vi "VI前面板截图.vi"(8 "矩形边界":T1 caption="子矩形", 11 "被绘图VI":refnum<vi>) -> (0 "错误输出":errorcluster, 2 "image subset":T2 caption="图像子集", 3 "new picture":picture caption="新图片")   [LabVIEW 2017]
doc: "获取VI截图或部分截图，矩形输入空则为全面版截图。"
uses:
  <vilib>/picture/picture.llb/imagedata.ctl
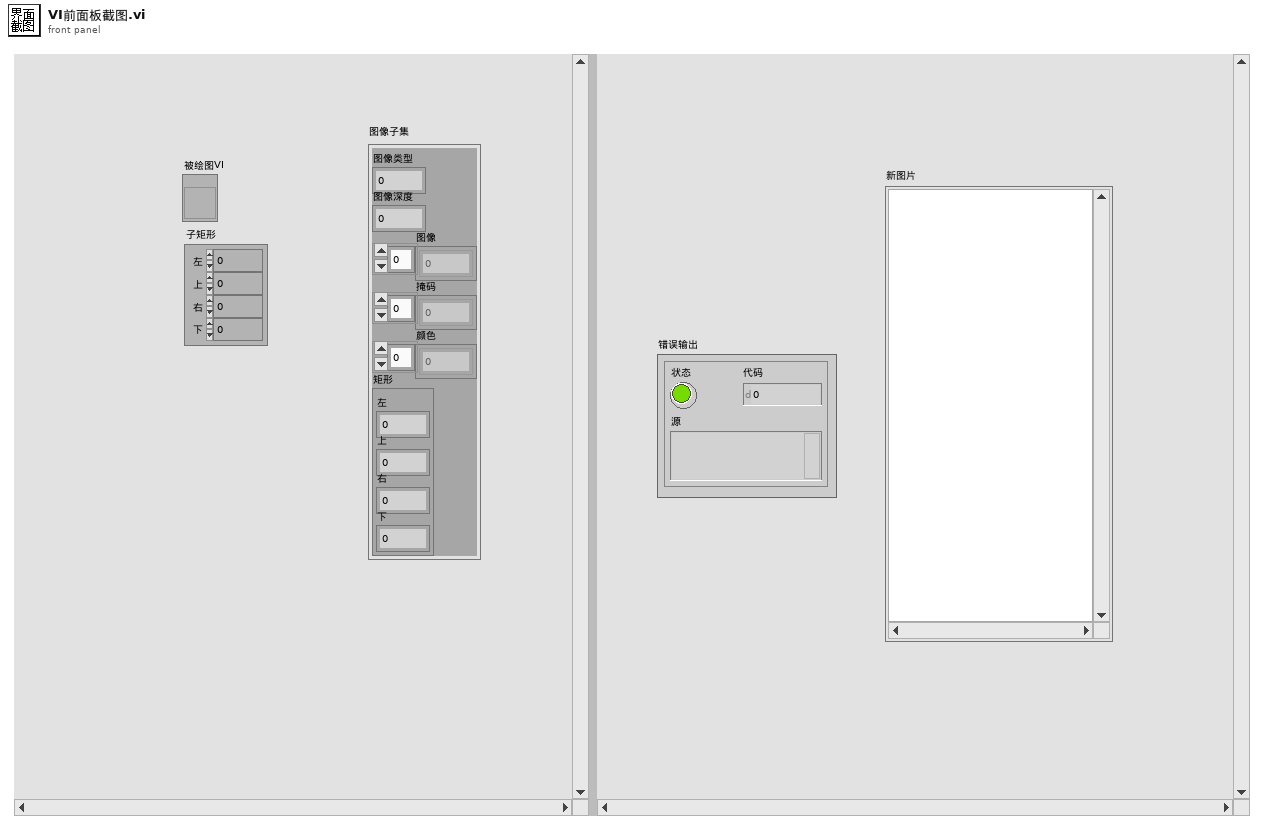
[diagram p1: front panel]
types:
  T1 = cluster{"left":i16, "top":i16, "right":i16, "bottom":i16}
  T2 = typedef "imagedata.ctl" = cluster{"image type":i32, "image depth":i32, "image":u8[], "mask":u8[], "colors":u32[], "Rectangle":cluster{"left":i16, "top":i16, "right":i16, "bottom":i16}}
  T3 = cluster{"left":bool, "top":bool, "right":bool, "bottom":bool}
  T4 = typedef "LVRectTypeDef.ctl" = cluster{"Left":i16, "Top":i16, "Right":i16, "Bottom":i16}
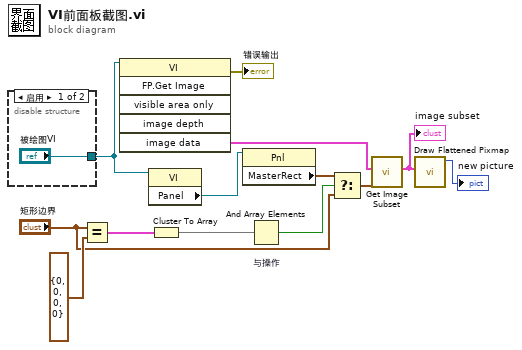
[diagram p0: block diagram]
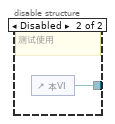
[diagram p2: hidden frame]
diagram:
  n1 = disable-structure shown="启用" {
    disable-tunnel: ["被绘图VI" w15] -> w6
    frame Enabled {
    }
    frame Disabled {
      # "测试使用"
      n2 = control-ref of="本VI"() -> (w15:refnum<vi>)
    }
  }
  n3 = Equal?(x="矩形边界", y=T1 {"left"=0, "top"=0, "right"=0, "bottom"=0} ("矩形边界")) -> (x = y?=w10:T3)
  n4 = invoke class="VI" method="FP.Get Image"(reference=w6) -> (error out=→"错误输出":errorcluster, "image data"=w13:T2)  [unwired: 5 in, 4 out]
  n5 = property class="VI"(reference=w6) -> ("Panel"=w5:refnum<vi>)  [unwired: 1 in, 2 out]
  n6 = Cluster To Array(cluster=w10) -> (array=w9:bool[])
  n7 = property class="Pnl"(reference=w5) -> ("MasterRect"=w3:T4)  [unwired: 1 in, 2 out]
  n8 = And Array Elements "与操作"(Boolean array=w9) -> (logical AND=w4:bool)
  n9 = Select(t=w3, s=w4, f="矩形边界") -> (s? t:f=w1:T4)
  n10 = call <vilib>:"Get Image Subset.vi"("subset rect"=w1, "image data"=w13) -> ("image subset"=w12:T2)  [unwired: 4 in, 1 out]
  "image subset" <- w12
  n11 = call <vilib>:"Draw Flattened Pixmap.vi"("image data"=w12) -> ("new picture"=→"new picture":picture)  [unwired: 8 in]
